vi "Menu-Start Acq.vi"(8 "error in":errorcluster, 11 "Menu in":refnum<k9>) -> ()   [LabVIEW 2016, in "CML UI.lvlib"]
uses:
  CML UI.lvlib
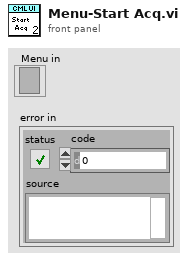
[diagram p1: front panel]
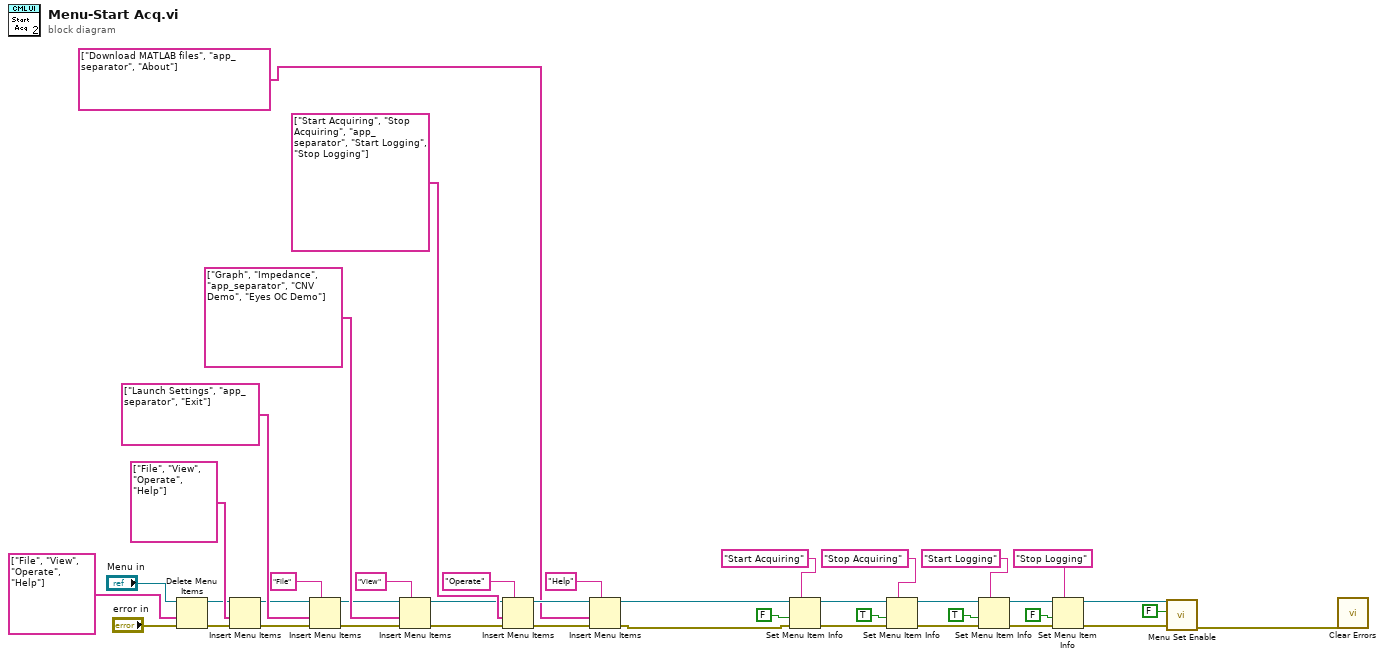
[diagram p0: block diagram]
diagram:
  n1 = Delete Menu Items(6:"error in", 7:string[] ["File", "View", "Operate", "Help"] ("L10n_item tags 1"), 9:"Menu in") -> (0:w20:errorcluster, 3:w21:refnum<k9>)  [unwired: 1 in]
  n2 = Insert Menu Items(6:w20, 7:string[] ["File", "View", "Operate", "Help"] ("L10n_item tags 1"), 9:w21) -> (0:w31:errorcluster, 3:w29:refnum<k9>)  [unwired: 3 in, 1 out]
  n3 = Insert Menu Items(5:"File" ("L10n_menu tag"), 6:w31, 7:string[] ["Launch Settings", "app_separator", "Exit"] ("L10n_item tags 2"), 9:w29) -> (0:w36:errorcluster, 3:w35:refnum<k9>)  [unwired: 2 in, 1 out]
  n4 = Insert Menu Items(5:"View" ("L10n_menu tag"), 6:w36, 7:string[] ["Graph", "Impedance", "app_separator", "CNV Demo", "Eyes OC Demo"] ("L10n_item tags 2"), 9:w35) -> (0:w40:errorcluster, 3:w39:refnum<k9>)  [unwired: 2 in, 1 out]
  n5 = Insert Menu Items(5:"Operate" ("L10n_menu tag"), 6:w40, 7:string[] ["Start Acquiring", "Stop Acquiring", "app_separator", "Start Logging", "Stop Logging"] ("L10n_item tags 2"), 9:w39) -> (0:w26:errorcluster, 3:w27:refnum<k9>)  [unwired: 2 in, 1 out]
  n6 = Insert Menu Items(5:"Help" ("L10n_menu tag"), 6:w26, 7:string[] ["Download MATLAB files", "app_separator", "About"] ("L10n_item tags 2"), 9:w27) -> (0:w24:errorcluster, 3:w25:refnum<k9>)  [unwired: 2 in, 1 out]
  n7 = Set Menu Item Info(7:"Start Acquiring" ("item tag"), 8:w24, 9:FALSE ("enabled"), 11:w25) -> (0:w6:errorcluster, 3:w7:refnum<k9>)  [unwired: 3 in]
  n8 = Set Menu Item Info(7:"Stop Acquiring" ("item tag"), 8:w6, 9:TRUE ("enabled"), 11:w7) -> (0:w14:errorcluster, 3:w15:refnum<k9>)  [unwired: 3 in]
  n9 = Set Menu Item Info(7:"Start Logging" ("item tag"), 8:w14, 9:TRUE ("enabled"), 11:w15) -> (0:w12:errorcluster, 3:w13:refnum<k9>)  [unwired: 3 in]
  n10 = Set Menu Item Info(7:"Stop Logging" ("item tag"), 8:w12, 9:FALSE ("enabled"), 11:w13) -> (0:w4:errorcluster, 3:w5:refnum<k9>)  [unwired: 3 in]
  n11 = call "Menu Set Enable.vi"("error in (no error)"=w4, "enabled ?"=FALSE, "Menu in"=w5) -> ("error out"=w3:errorcluster)  [unwired: 7 in, 1 out]
  n12 = call <vilib>:"Clear Errors.vi"("error in (no error)"=w3) -> ()  [unwired: 5 in, 2 out]
